vi "log_errors.vi"(1 "error in (no error)":errorcluster, 2 "dynamic data":T1) -> ()   [LabVIEW 2011]
uses:
  typedefs/dynamic_data.ctl
  <vilib>/vision/Image Controls.llb/IMAQ Image.ctl
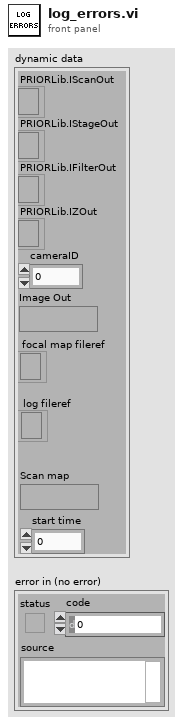
[diagram p1: front panel]
types:
  T1 = typedef "dynamic_data.ctl" = cluster{"PRIORLib.IScanOut":refnum<k7>, "PRIORLib.IStageOut":refnum<k7>, "PRIORLib.IFilterOut":refnum<k7>, "PRIORLib.IZOut":refnum<k7>, "cameraID":u32, "Image Out":T2, "focal map fileref":refnum<file>, "Scan map":T2, "start time":u32, "log fileref":refnum<file>}
  T2 = typedef "IMAQ Image.ctl" = refnum<image>
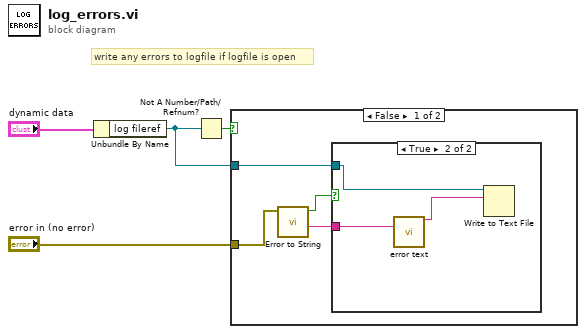
[diagram p0: block diagram]
diagram:
  # "write any errors to logfile if logfile is open"
  n1 = Unbundle By Name("dynamic data") -> ("log fileref"=w1:refnum<file>)
  n2 = Not A Number/Path/Refnum?(number/path/refnum=w1) -> (NaN/Path/Refnum?=w2:bool)
  n3 = case shown="False" w2 {
    tunnel: "error in (no error)" -> [w8 _]
    tunnel: w1 -> [w5 _]
    frame False {
      n4 = call "Error to String.vi"("Error In"=w8) -> ("Error String"=w6:string, "error status"=w7:bool)  [unwired: 5 in]
      n5 = case shown="True" w7 {
        tunnel: w6 -> [_ w11]
        tunnel: w5 -> [_ w9]
        frame False {
        }
        frame True {
          n6 = call "error text"("error"=w11) -> ("Result"=w10:string)  [unwired: 13 in, 1 out]
          n7 = Write to Text File(file (use dialog)=w9, text=w10) -> ()  [unwired: 2 in, 3 out]
        }
      }
    }
    frame True {
    }
  }
